vi "Periodic Tasks.vi"(8 "error in":errorcluster) -> ()   [LabVIEW 2016]
doc: "This VI runs in parallel to other tasks. It can contain as many user-defined periodic loops as you need. These can carry out PID or other sorts of timed response."
panel:
  out "error out":errorcluster
  out "Left Sensor Position":dbl
  out "Left Sensor Velocity":dbl
  out "Right Sensor Position":dbl
  out "Right Sensor Velocity":dbl
  out "Right Encoder Velocity":dbl
  out "Right Encoder Position":dbl
  out "Left Encoder Velocity":dbl
  out "Left Encoder Position":dbl
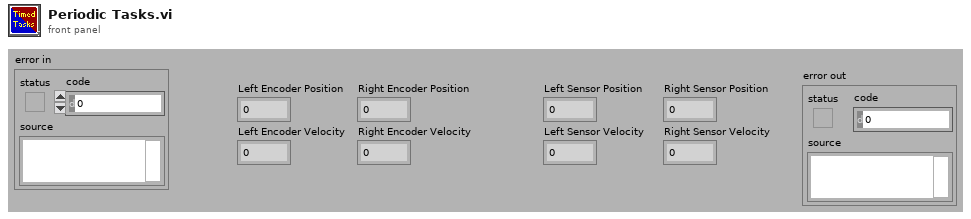
[diagram p1: front panel]
types:
  T1 = typedef "WPI_MotorControlDeviceRef.ctl" = cluster{"DeviceStatus":errorcluster, "Type":T2, "PWM":cluster{"PWM Channel":T3, "DeadBand":T4}, "CAN":cluster{"Device Number":u8, "SetOutput VI Ref":variant, "GetOutput VI Ref":variant, "Enable VI Ref":variant, "Disable VI Ref":variant, "Data":variant}, "Invert":bool}
  T2 = typedef "WPI_MotorControlType.ctl" = enum16{"PWM", "CAN"}
  T3 = typedef "FPGA_DIOPWMChannel.ctl" = enum8{"PWM 0", "PWM 1", "PWM 2", "PWM 3", "PWM 4", "PWM 5", "PWM 6", "PWM 7", "PWM 8", "PWM 9", "PWM MXP 0", "PWM MXP 1", "PWM MXP 2", "PWM MXP 3", "PWM MXP 4", "PWM MXP 5", "PWM MXP 6", "PWM MXP 7", "PWM MXP 8", "PWM MXP 9", "Invalid"}
  T4 = typedef "WPI_PWMDeadband.ctl" = cluster{"Name":string, "maxPositivePwm":i32, "minPositivePwm":i32, "centerPwm":i32, "maxNegativePwm":i32, "minNegativePwm":i32, "angularRange":u16}
  T5 = typedef "WPI_CANTalonSRX_GlobalStatus.ctl" = cluster{"Applied Throttle":dbl, "Module Enabled":bool, "CAN Error":errorcluster, "Closed Loop Error":dbl, "Forward Limit Switch Closed":bool, "Reverse Limit Switch Closed":bool, "Sensor Position":dbl, "Sensor Velocity":dbl, "Current":dbl, "Sticky Fault - Over Temp":bool, "Sticky Fault - Under Voltage":bool, "Sticky Fault - Forward Limit":bool, "Sticky Fault - Reverse Limit":bool, "Sticky Fault - Forward Soft Limit":bool, "Sticky Fault - Reverse Soft Limit":bool, "Brake is Enabled":bool, "Encoder Position":dbl, "Encoder Velocity":dbl, "Encoder Index Count":dbl, "Encoder A Pin State":bool, "Encoder B Pin State":bool, "Encoder Index Pin State":bool, "Analog In":dbl, "Analog In Velocity":dbl, "Temperature (C)":dbl, "Battery Voltage":dbl, "Control 5 Is Supported":bool, "Current Profile Slot Select":dbl, "Pos Div 8":bool, "Vel Div 4":bool, "Pulse Width Position":i32, "Pulse Width Velocity":i32, "Pulse Width Rise To Rise (us)":i32, "Pulse Width Rise To Fall (us)":i32, "Mot Prof Active Is Under Run":bool, "Mot Prof Active Has Under Run":bool, "Mot Prof Active Is Last":bool, "Mot Prof Active Velocity Only":bool, "Mot Prof Active Is Valid":bool, "Mot Prof Buffer Is Full":bool, "Mot Prof Active Profile Slot Select":i32, "Mot Prof NextID":i32, "Mot Prof Count":i32, "Mot Prof Active Velocity":dbl, "Mot Prof Active Position":dbl, "Mot Prof Output Enable":i32}
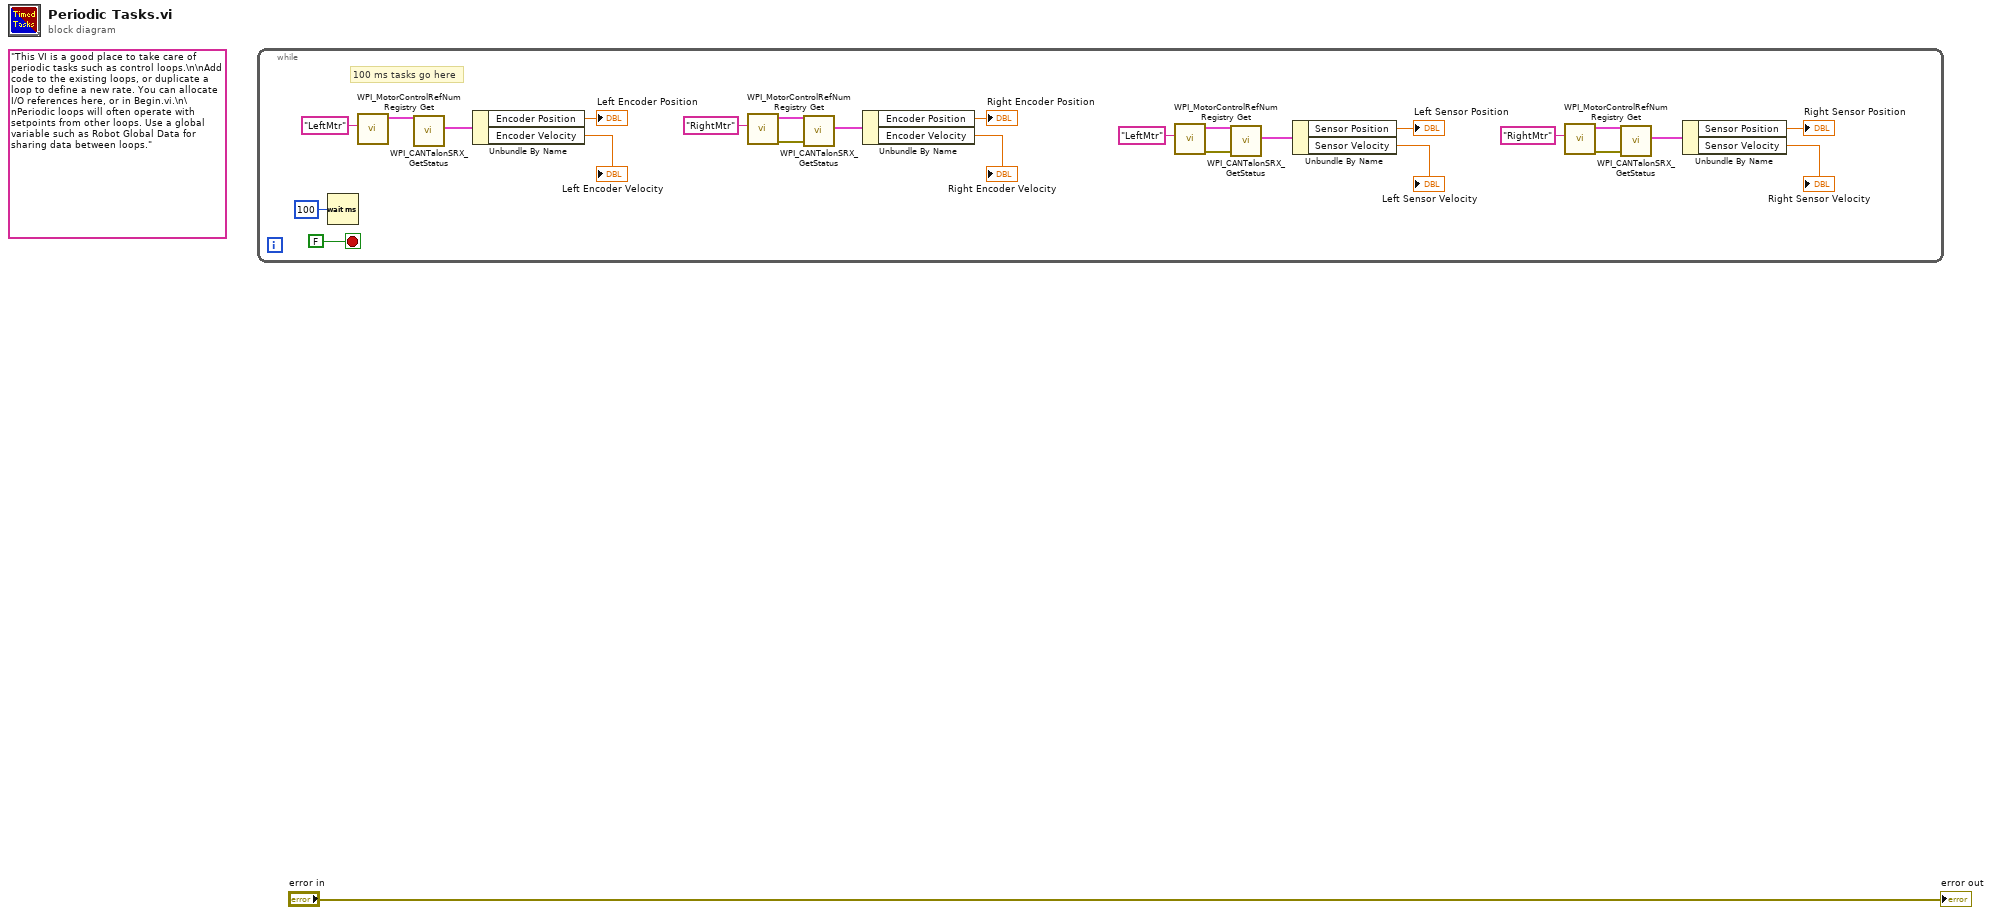
[diagram p0: block diagram]
diagram:
  (unwired) "This VI is a good place to take care of periodic tasks such as control loops.\n\nAdd code to the existing loops, or duplicate a loop to define a new rate. You can allocate I/O references here, or in Begin.vi.\n\nPeriodic loops will often operate with setpoints from other loops. Use a global variable such as Robot Global Data for sharing data between loops."
  n1 = while {
    stop <- FALSE stop-if-true
    # "100 ms tasks go here"
    n2 = Wait (ms)(milliseconds to wait=u32 100) -> ()  [unwired: 1 out]
    n3 = call <vilib>:"WPI_MotorControlRefNum Registry Get.vi"("refnum name"="LeftMtr") -> ("MotorControlDevRef"=w20:T1)  [unwired: 9 in, 1 out]
    n4 = call <vilib>:"WPI_CANTalonSRX_GetStatus.vi"("CAN Talon SRX Ref"=w20) -> ("Talon SRX Status"=w18:T5)  [unwired: 8 in, 2 out]
    n5 = Unbundle By Name(w18) -> ("Encoder Position"=→"Left Encoder Position":dbl, "Encoder Velocity"=→"Left Encoder Velocity":dbl)
    n6 = call <vilib>:"WPI_MotorControlRefNum Registry Get.vi"("refnum name"="RightMtr") -> ("error out"=w12:errorcluster, "MotorControlDevRef"=w13:T1)  [unwired: 9 in]
    n7 = call <vilib>:"WPI_CANTalonSRX_GetStatus.vi"("error in (no error)"=w12, "CAN Talon SRX Ref"=w13) -> ("Talon SRX Status"=w15:T5)  [unwired: 7 in, 2 out]
    n8 = Unbundle By Name(w15) -> ("Encoder Position"=→"Right Encoder Position":dbl, "Encoder Velocity"=→"Right Encoder Velocity":dbl)
    n9 = call <vilib>:"WPI_MotorControlRefNum Registry Get.vi"("refnum name"="LeftMtr") -> ("error out"=w2:errorcluster, "MotorControlDevRef"=w3:T1)  [unwired: 9 in]
    n10 = call <vilib>:"WPI_CANTalonSRX_GetStatus.vi"("error in (no error)"=w2, "CAN Talon SRX Ref"=w3) -> ("Talon SRX Status"=w5:T5)  [unwired: 7 in, 2 out]
    n11 = Unbundle By Name(w5) -> ("Sensor Position"=→"Left Sensor Position":dbl, "Sensor Velocity"=→"Left Sensor Velocity":dbl)
    n12 = call <vilib>:"WPI_MotorControlRefNum Registry Get.vi"("refnum name"="RightMtr") -> ("error out"=w11:errorcluster, "MotorControlDevRef"=w10:T1)  [unwired: 9 in]
    n13 = call <vilib>:"WPI_CANTalonSRX_GetStatus.vi"("error in (no error)"=w11, "CAN Talon SRX Ref"=w10) -> ("Talon SRX Status"=w8:T5)  [unwired: 7 in, 2 out]
    n14 = Unbundle By Name(w8) -> ("Sensor Position"=→"Right Sensor Position":dbl, "Sensor Velocity"=→"Right Sensor Velocity":dbl)
  }
  "error out" <- "error in"
